vi "Create PPL Migrator.vi"(0 "Project Refnum":refnum<vi>, 5 "Plug-in name":string, 7 "Main VI Name":string, 9 "Library name":string, 11 "error in (no error)":errorcluster) -> (4 "project ref out":refnum<vi>, 6 "path":path, 15 "error out":errorcluster)   [LabVIEW 2021, in "NI_AB_API_PPL_Extensions.lvclass"]
uses:
  NI_AB_API_PPL_Extensions.lvclass
  G Plugin Editor.lvlib
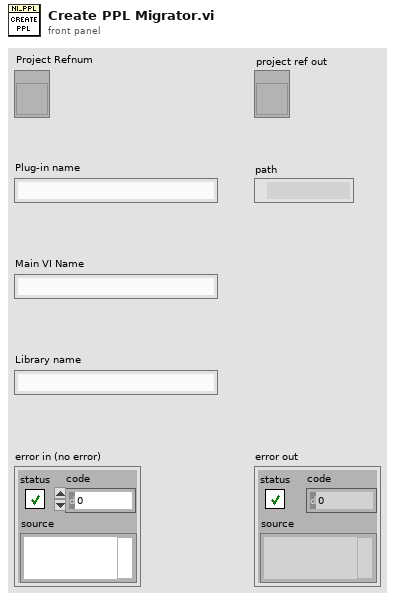
[diagram p1: front panel]
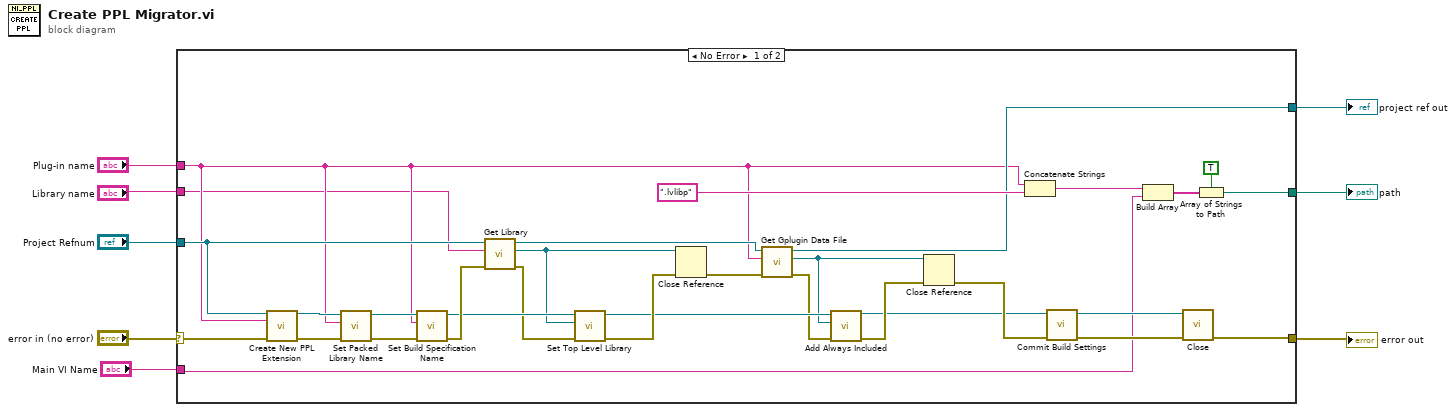
[diagram p0: block diagram]
diagram:
  n1 = case shown="No Error" "error in (no error)" {
    selector: "error in (no error)" -> [w39 w41]
    tunnel: [w28 w41] -> w8
    tunnel: "Project Refnum" -> [w38 w40]
    tunnel: "Plug-in name" -> [w18 _]
    tunnel: [w19 w40] -> w4
    tunnel: [w25 _] -> w3
    tunnel: "Library name" -> [w10 _]
    tunnel: "Main VI Name" -> [w9 _]
    frame No Error {
      n2 = call "Create New PPL Extension.vi"("Project Refnum"=w38, "Build specification name"=w18, "error in (no error)"=w39) -> ("NI_AB_API_Build out"=w24:refnum<class "NI_AB_API_PPL_Extensions.lvclass">, "error out"=w21:errorcluster)  [unwired: 11 in]
      n3 = call-dynamic "Set Packed Library Name.vi"("error in (no error)"=w21, "Packed library name"=w18, "PPL in"=w24) -> ("error out"=w22:errorcluster, "PPL out"=w23:refnum<class "NI_AB_API_PPL_Extensions.lvclass">)  [unwired: 7 in]
      n4 = call-dynamic "Set Build Specification Name.vi"("error in (no error)"=w22, "Build Specification Name"=w18, "NI_AB_API_PPL in"=w23) -> ("error out"=w37:errorcluster, "NI_AB_API_PPL out"=w36:refnum<class "NI_AB_API_PPL_Extensions.lvclass">)  [unwired: 7 in]
      n5 = call "Get Library.vi"("error in (no error)"=w37, "library name"=w10, "project ref"=w38) -> ("error out"=w35:errorcluster, "library item"=w29:refnum<vi>, "project ref out"=w20:refnum<vi>)  [unwired: 5 in, 1 out]
      n6 = call-dynamic "Set Top Level Library.vi"("error in (no error)"=w35, "ProjectItem Refnum"=w29, "PPL in"=w36) -> ("error out"=w33:errorcluster, "PPL out"=w17:refnum<class "NI_AB_API_PPL_Extensions.lvclass">)  [unwired: 7 in]
      n7 = Close Reference(reference=w29, error in (no error)=w33) -> (error out=w11:errorcluster)
      n8 = call "Get Gplugin Data File.vi"("error in (no error)"=w11, "library name"=w18, "project ref"=w20) -> ("error out"=w12:errorcluster, "Document item"=w16:refnum<vi>, "project ref out"=w19:refnum<vi>)  [unwired: 5 in, 1 out]
      n9 = call-dynamic "Add Always Included.vi"("error in (no error)"=w12, "ProjectItem Refnum"=w16, "PPL in"=w17) -> ("error out"=w15:errorcluster, "PPL out"=w13:refnum<class "NI_AB_API_PPL_Extensions.lvclass">)  [unwired: 7 in]
      n10 = Close Reference(reference=w16, error in (no error)=w15) -> (error out=w14:errorcluster)
      n11 = Concatenate Strings(w18, ".lvlibp" ("string")) -> (w31:string)
      n12 = call-dynamic "Commit Build Settings.vi"("error in (no error)"=w14, "PPL in"=w13) -> ("error out"=w34:errorcluster, "PPL out"=w30:refnum<class "NI_AB_API_PPL_Extensions.lvclass">)  [unwired: 8 in]
      n13 = Build Array(w31, w9) -> (w26:string[])
      n14 = call-dynamic "Close.vi"("error in (no error)"=w34, "DLL in"=w30) -> ("error out"=w28:errorcluster)  [unwired: 9 in]
      n15 = Array of Strings to Path(0:w26, 1:TRUE ("relative")) -> (2:w25:path)
    }
    frame Error {
    }
  }
  "error out" <- w8
  "project ref out" <- w4
  "path" <- w3
